vi "Check Subnet.vi"(9 "Mask":u32 format="%.0x", 10 "Address 2":u32 format="%.0x", 11 "Address 1":u32 format="%.0x") -> (3 "In Subnet":bool)   [LabVIEW 2021, in "Networking_CIF_U.lvlib"]
uses:
  Networking_CIF_U.lvlib
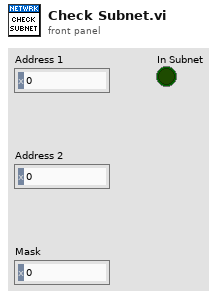
[diagram p1: front panel]
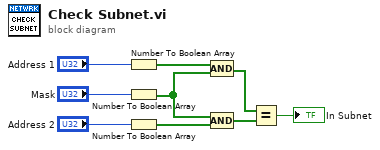
[diagram p0: block diagram]
diagram:
  n1 = Number To Boolean Array(number="Address 1") -> (Boolean array=w6:bool[])
  n2 = Number To Boolean Array(number="Mask") -> (Boolean array=w4:bool[])
  n3 = Number To Boolean Array(number="Address 2") -> (Boolean array=w5:bool[])
  n4 = Compound Arithmetic op=AND(w6, w4) -> (w2:bool[])
  n5 = Compound Arithmetic op=AND(w4, w5) -> (w3:bool[])
  n6 = Equal?(x=w2, y=w3) -> (x = y?=→"In Subnet":bool)
